vi "Fetch Excel (xlsx).vi"(6 "columns (21)":i32=21, 7 "Excel._SheetName":string="Sheet1", 8 "error in (no error)":errorcluster, 11 "excelRefs in":T1) -> (0 "error out":errorcluster, 2 "data":string[][](array[string]), 3 "excelRefs out":T1)   [LabVIEW 2020]
uses:
  Controls/excelRefContainer.ctl
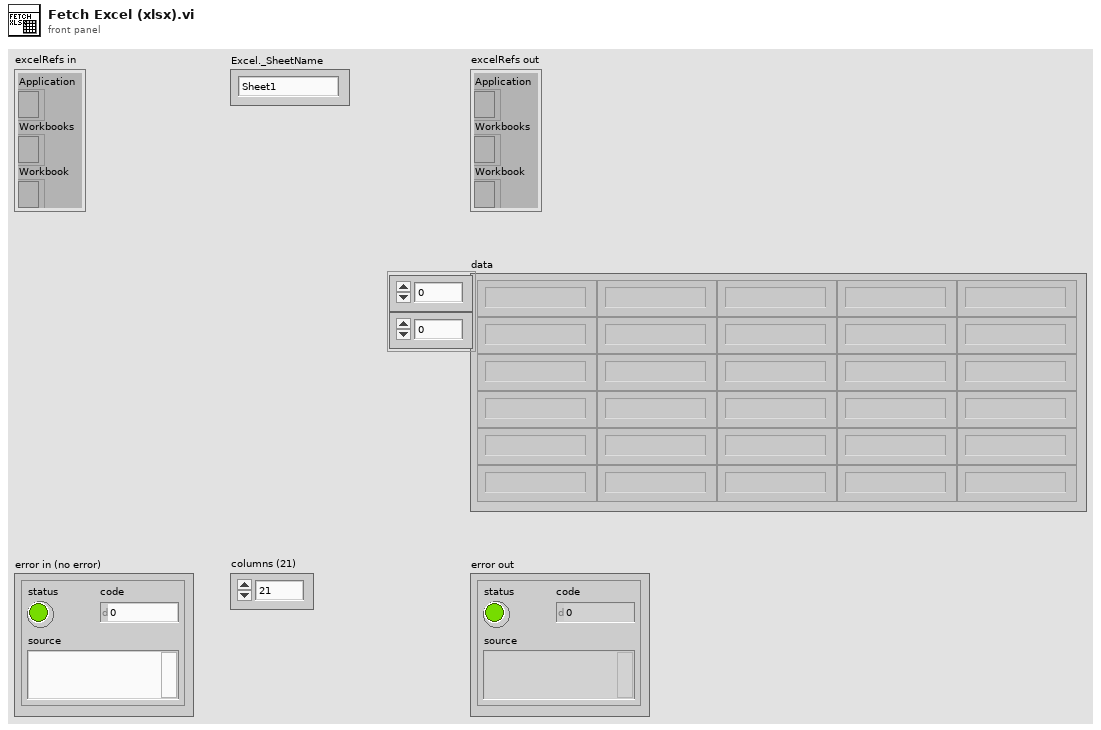
[diagram p1: front panel]
types:
  T1 = typedef "excelRefContainer.ctl" = cluster{"Application":refnum<k7>, "Workbooks":refnum<k7>, "Workbook":refnum<k7>}
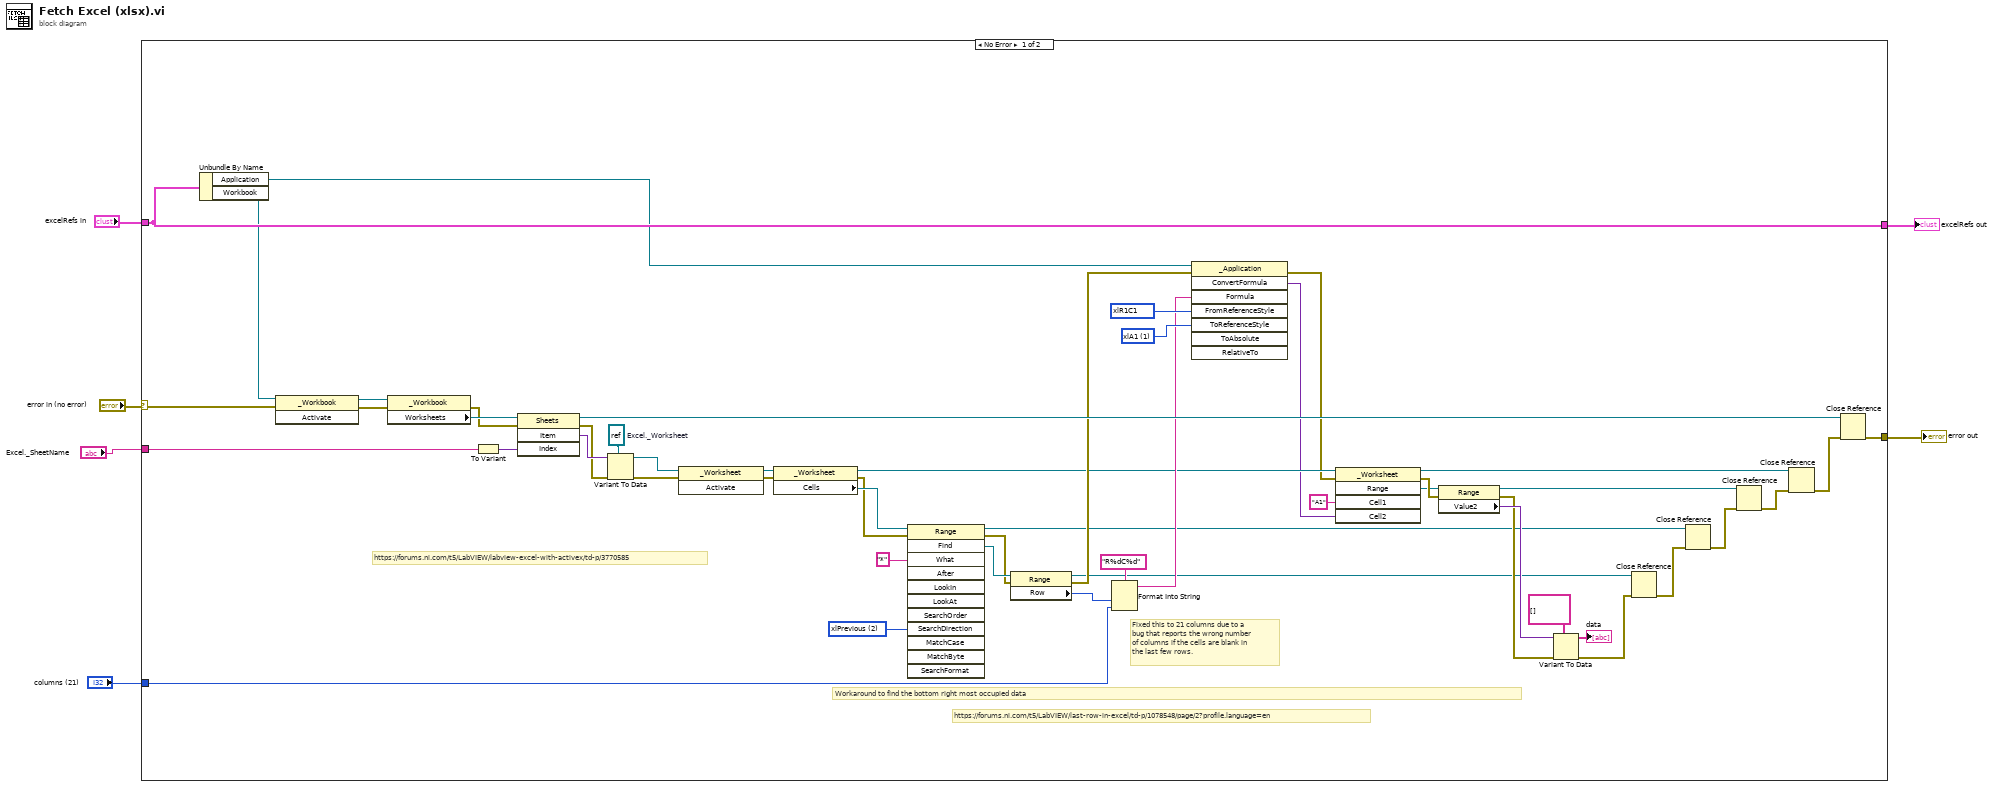
[diagram p0: block diagram]
diagram:
  n1 = case shown="No Error" "error in (no error)" {
    selector: "error in (no error)" -> [w12 w58]
    tunnel: [w13 w58] -> w6
    tunnel: [w11 w59] -> w5
    tunnel: "excelRefs in" -> [w11 w59]
    tunnel: "Excel._SheetName" -> [w8 _]
    tunnel: "columns (21)" -> [w7 _]
    frame No Error {
      w34 = 1 items=["xlA1"=1, "xlR1C1"=-4150] ("FromReferenceStyle")
      w35 = -4150 items=["xlA1"=1, "xlR1C1"=-4150] ("FromReferenceStyle")
      w39 = 2 items=["xlNext"=1, "xlPrevious"=2] ("SearchDirection")
      w54 = refnum<k7> refnum  # Excel._Worksheet
      # "Fixed this to 21 columns due to a bug that reports the wrong number of columns if the cells are blank in the last few rows."
      # "https://forums.ni.com/t5/LabVIEW/last-row-in-excel/td-p/1078548/page/2?profile.language=en"
      # "Workaround to find the bottom right most occupied data"
      # "https://forums.ni.com/t5/LabVIEW/labview-excel-with-activex/td-p/3770585"
      n2 = Unbundle By Name(w11) -> ("Application"=w9:refnum<k7>, "Workbook"=w10:refnum<k7>)
      n3 = invoke class="_Workbook" method="Activate"(reference=w10, error in=w12) -> (reference out=w57:refnum<k7>, error out=w53:errorcluster)  [unwired: 1 in, 1 out]
      n4 = property class="_Workbook"(reference=w57, error in=w53) -> (error out=w29:errorcluster, "Worksheets"=w43:refnum<k7>)  [unwired: 1 out]
      n5 = To Variant(anything=w8) -> (Variant=w56:variant)
      n6 = invoke class="Sheets" method="Item"(reference=w43, error in=w29, "Index"=w56) -> (reference out=w44:refnum<k7>, error out=w52:errorcluster, "Item"=w55:variant)  [unwired: 1 in, 1 out]
      n7 = Variant To Data(error in=w52, type=w54, Variant=w55) -> (data=w51:refnum<k7>, error out=w50:errorcluster)
      n8 = invoke class="_Worksheet" method="Activate"(reference=w51, error in=w50) -> (reference out=w46:refnum<k7>, error out=w45:errorcluster)  [unwired: 1 in, 1 out]
      n9 = property class="_Worksheet"(reference=w46, error in=w45) -> (reference out=w27:refnum<k7>, error out=w41:errorcluster, "Cells"=w42:refnum<k7>)
      n10 = invoke class="Range" method="Find"(reference=w42, error in=w41, "What"="*", "SearchDirection"=w39) -> (reference out=w20:refnum<k7>, error out=w31:errorcluster, "Find"=w38:refnum<k7>)  [unwired: 8 in, 9 out]
      n11 = property class="Range"(reference=w38, error in=w31) -> (reference out=w16:refnum<k7>, error out=w28:errorcluster, "Row"=w36:i32)
      n12 = Format Into String(format string="R%dC%d", w36, w7) -> (resulting string=w30:string)  [unwired: 2 in, 1 out]
      n13 = invoke class="_Application" method="ConvertFormula"(reference=w9, error in=w28, "Formula"=w30, "FromReferenceStyle"=w35, "ToReferenceStyle"=w34) -> (error out=w24:errorcluster, "ConvertFormula"=w25:variant)  [unwired: 3 in, 6 out]
      n14 = invoke class="_Worksheet" method="Range"(reference=w27, error in=w24, "Cell1"="A1" ("format string"), "Cell2"=w25) -> (reference out=w26:refnum<k7>, error out=w23:errorcluster, "Range"=w22:refnum<k7>)  [unwired: 1 in, 2 out]
      n15 = property class="Range"(reference=w22, error in=w23) -> (reference out=w17:refnum<k7>, error out=w21:errorcluster, "Value2"=w32:variant)
      n16 = Variant To Data(error in=w21, type=string[][] [], Variant=w32) -> (data=→"data":string[][], error out=w15:errorcluster)
      n17 = Close Reference(reference=w16, error in (no error)=w15) -> (error out=w14:errorcluster)
      n18 = Close Reference(reference=w20, error in (no error)=w14) -> (error out=w19:errorcluster)
      n19 = Close Reference(reference=w17, error in (no error)=w19) -> (error out=w18:errorcluster)
      n20 = Close Reference(reference=w26, error in (no error)=w18) -> (error out=w47:errorcluster)
      n21 = Close Reference(reference=w44, error in (no error)=w47) -> (error out=w13:errorcluster)
    }
    frame Error {
    }
  }
  "error out" <- w6
  "excelRefs out" <- w5
